vi "THzTime_SPEED_control_TA_170214.vi"(1 "ESP300 Axis":i8=1, 2 "ESP300 Address":string="1", 4 "Lockin Address":string="12") -> ()   [LabVIEW 2010]
panel:
  in  "Axis 1 Step btw Pos":dbl=0.1
  in  "Delay":u32=1500
  in  "?":bool
  in  "# of Avg":i32=8
  in  "Axis 1 # of Pos":u16=40
  in  "Axis 1 Starting Pos":dbl=14.5
  in  "SHOT202 Address":string="8"
  out "Y position":dbl=-0.2690666666666667 format="%#.3p"
  out "X position":dbl=-0.49996666666666667 format="%#.3p"
  out "Power meter":dbl=48.71333333333333 format="%#.3p"
  in  "Save File Name":string="bc_"
  in  "Launch server?":bool
  in  "Authorize?":bool=TRUE
  in  "CONEX-PSD9 Instrument Key 2":string="CONEX-PSD (A6ULD73M)"
  in  "Interdelay (ms)":dbl=20.0
  in  "pre delay(ms)":dbl=300.0
  out "Lock-in Y-Channel":dbl=3.63801e-12 format="%#.3p"
  out "Lock-in X-Channel":dbl=-3.4561e-11 format="%#.3p"
  out "THz Time-domain Signal Wave":cluster{"x-axis":sgl[], "y-axis":dbl[]}(graph)={"x-axis"=[-14.5, -14.51, -14.52, -14.53, -14.54, -14.55, -14.56, -14.57, -14.58, -14.59, -14.6, -14.61], "y-axis"=[1.819e-12, 1.819e-12, 0.0, 0.0, -1.819e-12, -7.27601e-12, -9.095e-12, -1.0914e-11, -1.6371e-11, -2.0009e-11, -2.1828e-11, -2.91041e-11]}
  in  "Autosave Directory for Long-term Average Scan":path=path "D:/taianh/Measurement Data/170219 Beam Calibration"
  in  "OK Button":bool
  out "Data Type":string="outp ? 1"
  in  "Enum":enum16{"X", "Y", "Abs"}(ring)
  in  "Draw":bool
  in  "Exit Program":bool
  in  "Short term \nAverage#":i8=1
  in  "Step":sgl=0.005 min=0 max=10000 format="%.3f"
  in  "End Position":sgl=-8.0 min=-75 max=75 format="%#.3f"
  in  "Start Position":sgl=-6.5 min=-75 max=75 format="%#.3f"
  # "THz Experiment"
  # "Data"
  # "Auto-offset"
  # "Start Position (mm)"
  # "End Position (mm)"
  # "Step (mm)"
  # "Point Avg"
  # "# of Avg"
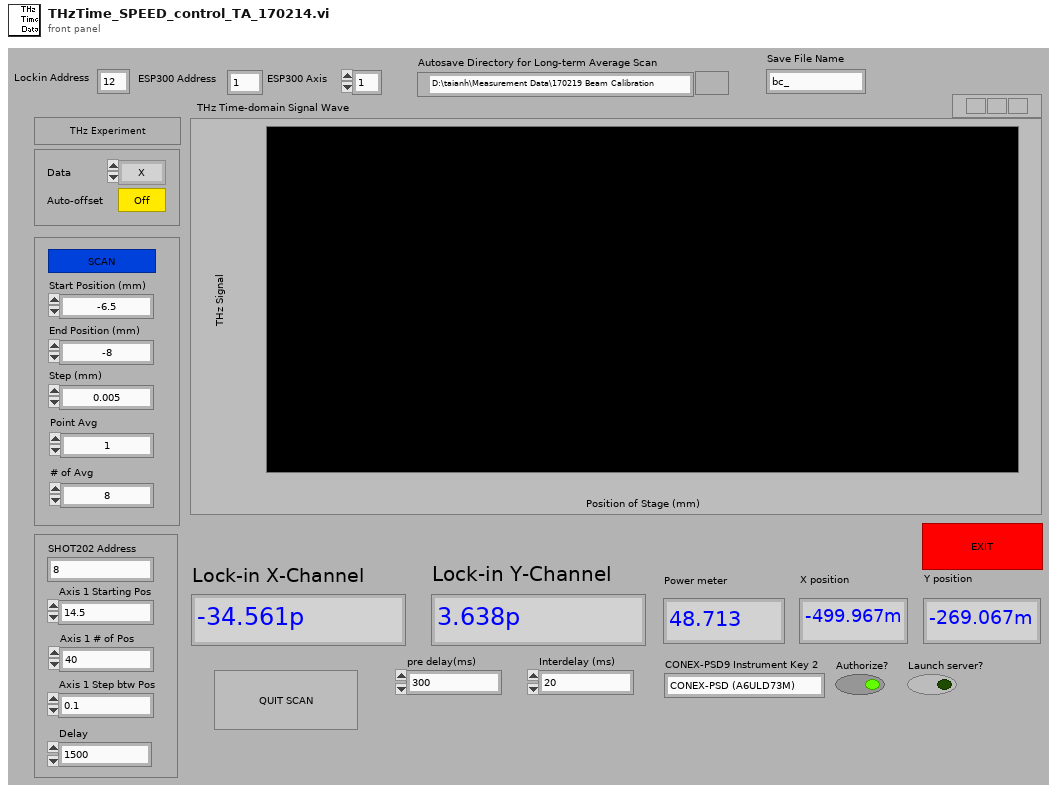
[diagram p1: front panel]
types:
  T1 = cluster{"ConexPSD Reference":refnum<k24>, "error out":errorcluster, "Component ID":i32}
  T2 = cluster{"Step Number":i32, "Step":sgl, "Start Position":sgl, "Time-out":i32, "Lockin Address":string, "Short term \nAverage#":i8, i32, "ESP300 Axis":i8, "Value":string, "pre delay(ms)":dbl, "Interdelay (ms)":dbl, "Autosave Directory for Long-term Average Scan":path, cluster{"ConexPSD Reference":refnum<k24>, "error out":errorcluster, "Component ID":i32}}
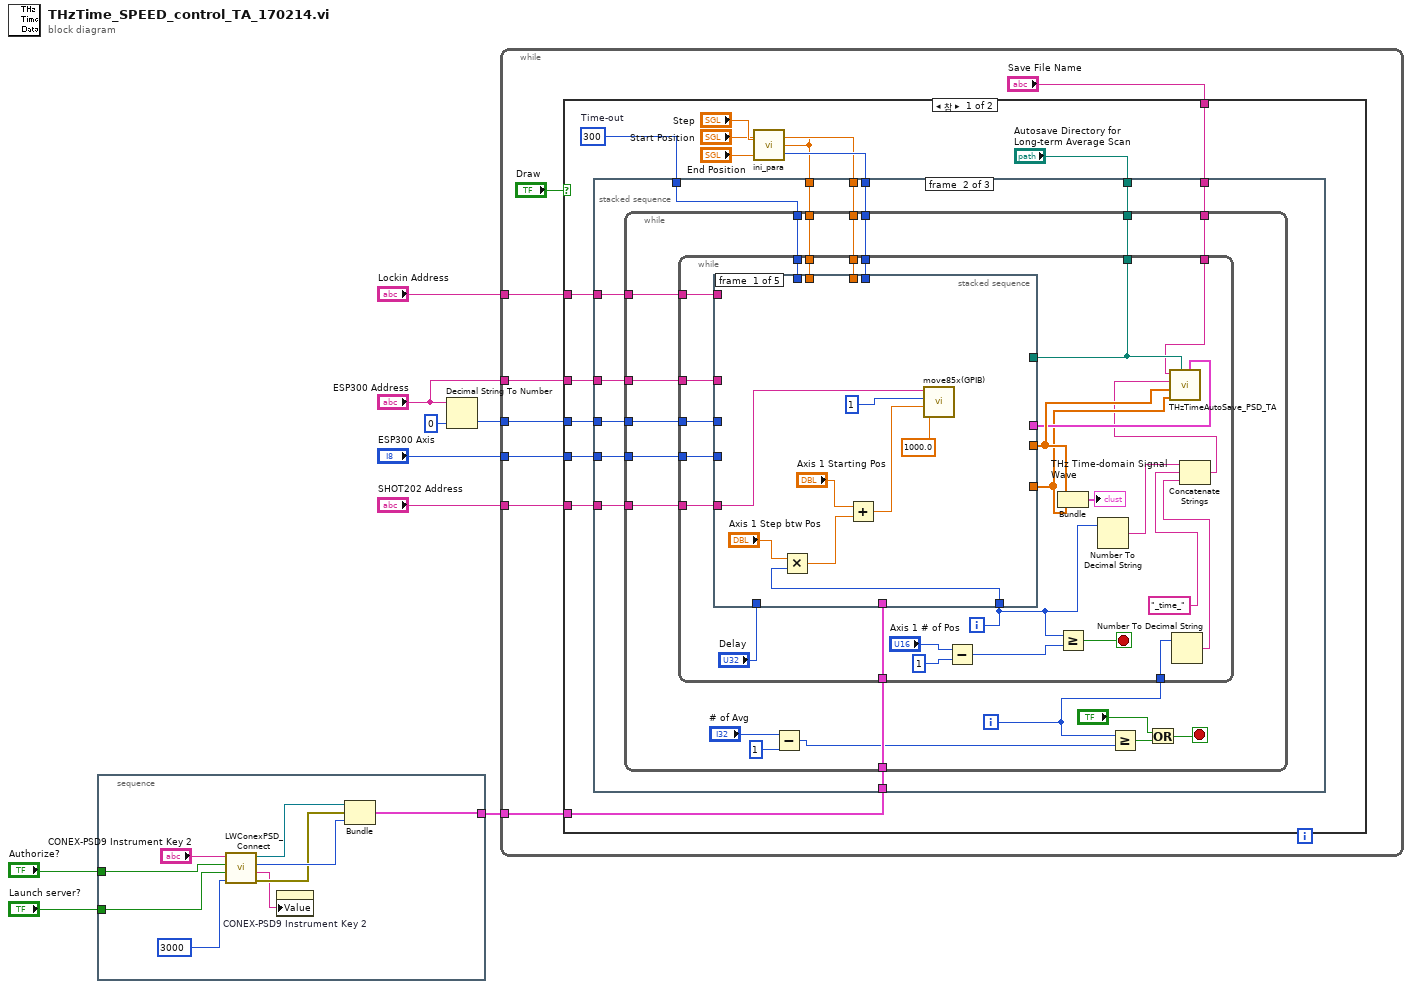
[diagram p0: block diagram]
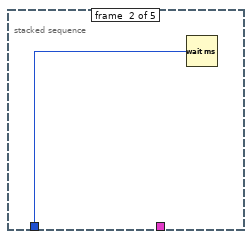
[diagram p3: hidden frame]
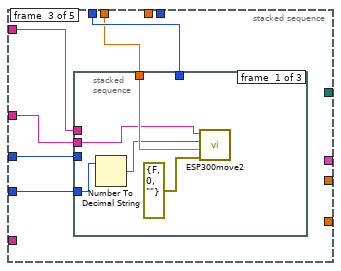
[diagram p4: hidden frame]
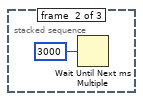
[diagram p5: hidden frame]
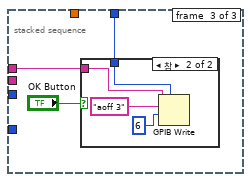
[diagram p6: hidden frame]
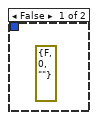
[diagram p7: hidden frame]
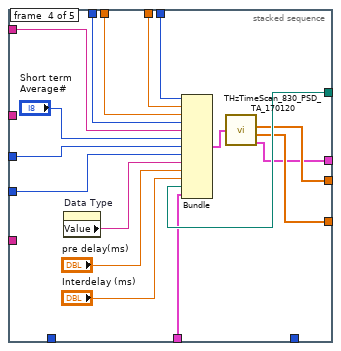
[diagram p8: hidden frame]
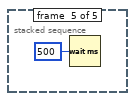
[diagram p9: hidden frame]
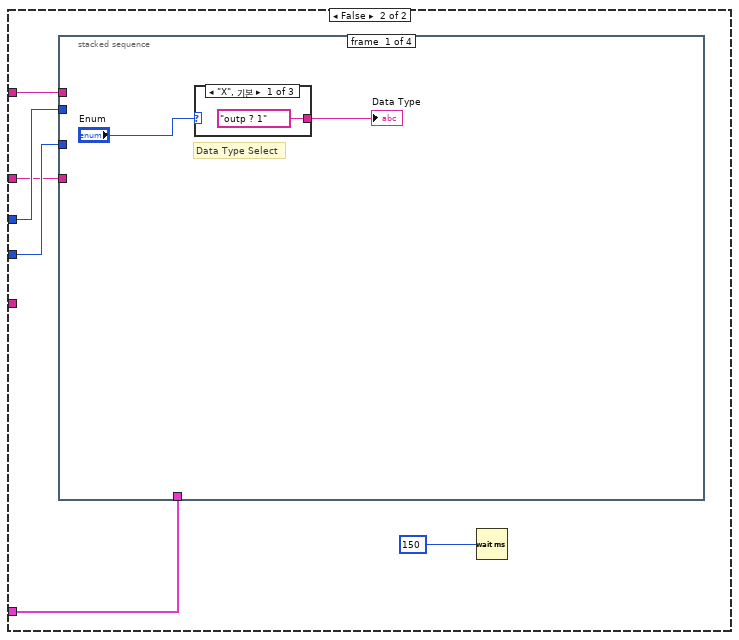
[diagram p11: hidden frame]
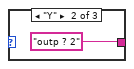
[diagram p12: hidden frame]
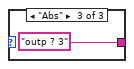
[diagram p13: hidden frame]
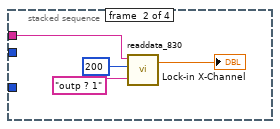
[diagram p14: hidden frame]
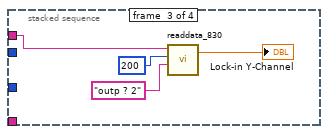
[diagram p15: hidden frame]
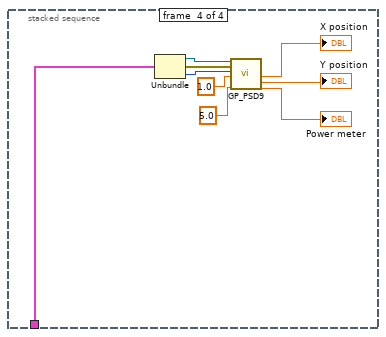
[diagram p16: hidden frame]
diagram:
  n1 = stacked-sequence {
    tunnel: "Authorize?" -> [w12]
    tunnel: [w11] -> w2
    tunnel: "Launch server?" -> [w10]
    frame #0 {
      n2 = call "LWConexPSD_Connect.vi"("DiscoverTimeout (10000 msec)"=3000, "Launch server? (True)"=w10, "Authorize? (True)"=w12, "Instrument Key"="CONEX-PSD9 Instrument Key 2") -> ("error out"=w16:errorcluster, "Instrument Key out"=w14:string, "Component ID"=w17:i32, "ConexPSD Reference"=w15:refnum<k24>)
      n3 = property on="CONEX-PSD9 Instrument Key 2" class="Str"("Value"=w14) -> ()  [unwired: 2 in, 2 out]
      n4 = Bundle("ConexPSD Reference"=w15, "error out"=w16, "Component ID"=w17) -> (w11:T1)  [unwired: 1 in]
    }
  }
  n5 = Decimal String To Number(string="ESP300 Address", default (0L)=0 ("default (0 I32)")) -> (number=w7:i32)  [unwired: 1 in, 1 out]
  n6 = while {
    tunnel: "ESP300 Axis" -> [w25]
    tunnel: "Lockin Address" -> [w24]
    tunnel: w7 -> [w23]
    tunnel: "ESP300 Address" -> [w22]
    tunnel: w2 -> [w21]
    tunnel: "SHOT202 Address" -> [w19]
    stop <- "Exit Program" stop-if-true
    n7 = case shown="참" "Draw" {
      tunnel: w24 -> [w41 w149]
      tunnel: w25 -> [w40 w151]
      tunnel: w23 -> [w39 w150]
      tunnel: w22 -> [w31 w147]
      tunnel: w21 -> [w30 w146]
      tunnel: "Save File Name" -> [w29 _]
      tunnel: w19 -> [w28 _]
      frame True {
        w38 = 300  # Time-out
        n8 = call "ini_para.vi"("End Position"="End Position", "Start Position"="Start Position", "Step"="Step") -> ("Step Number"=w35:i32, "Step"=w34:sgl)
        n9 = stacked-sequence {
          tunnel: w41 -> [_ w53 _]
          tunnel: w38 -> [_ w52 _]
          tunnel: w40 -> [_ w51 _]
          tunnel: w39 -> [_ w50 _]
          tunnel: w35 -> [_ w48 _]
          tunnel: w34 -> [_ w46 _]
          tunnel: "Start Position" -> [_ w49 _]
          tunnel: "Autosave Directory for Long-term Average Scan" -> [_ w47 _]
          tunnel: w31 -> [_ w45 _]
          tunnel: w30 -> [_ w44 _]
          tunnel: w29 -> [_ w43 _]
          tunnel: w28 -> [_ w42 _]
          frame #0 {
          }
          frame #1 {
            n10 = while {
              tunnel: w53 -> [w72]
              tunnel: w52 -> [w71]
              tunnel: w51 -> [w70]
              tunnel: w50 -> [w69]
              tunnel: w49 -> [w68]
              tunnel: w48 -> [w67]
              tunnel: w47 -> [w66]
              tunnel: w46 -> [w65]
              tunnel: w45 -> [w64]
              tunnel: w44 -> [w63]
              tunnel: w43 -> [w62]
              tunnel: w42 -> [w61]
              i -> [w54]
              stop <- w56 stop-if-true
              n11 = while {
                tunnel: w71 -> [w98]
                tunnel: w72 -> [w99]
                tunnel: w70 -> [w97]
                tunnel: w69 -> [w96]
                tunnel: w68 -> [w95]
                tunnel: w65 -> [w94]
                tunnel: w67 -> [w93]
                tunnel: w66 -> [w88]
                tunnel: w64 -> [w91]
                tunnel: w63 -> [w90]
                tunnel: w62 -> [w87]
                tunnel: w61 -> [w84]
                tunnel: w54 -> [w75]
                i -> [w78]
                stop <- w83 stop-if-true
                n12 = stacked-sequence {
                  tunnel: w99 -> [_ _ w114 w140 _]
                  tunnel: w98 -> [_ _ w113 w141 _]
                  tunnel: w97 -> [_ _ w112 w137 _]
                  tunnel: w96 -> [_ _ w111 w138 _]
                  tunnel: w95 -> [_ _ w110 w142 _]
                  tunnel: w94 -> [_ _ _ w143 _]
                  tunnel: w93 -> [_ _ _ w144 _]
                  tunnel: [_ _ _ w131 _] -> w89
                  tunnel: [_ _ _ w130 _] -> w85
                  tunnel: w91 -> [_ _ w109 _ _]
                  tunnel: w88 -> [_ _ _ w133 _]
                  tunnel: w90 -> [_ _ _ w132 _]
                  tunnel: [_ _ _ w129 _] -> w86
                  tunnel: w84 -> [w107 _ _ _ _]
                  tunnel: w78 -> [w105 _ _ _ _]
                  tunnel: "Delay" -> [_ w108 _ _ _]
                  frame #0 {
                    n13 = Multiply(x="Axis 1 Step btw Pos", y=w105) -> (x*y=w102:dbl)
                    n14 = Add(x="Axis 1 Starting Pos", y=w102) -> (x+y=w101:dbl)
                    n15 = call "move85x(GPIB).vi"("wait time(ms)"=1000.0, "Moving Distance (mm) : resolutino is 1um"=w101, "Axis Number"=u8 1, "SHOT202 Address"=w107) -> ()
                  }
                  frame #1 {
                    n16 = Wait (ms)(milliseconds to wait=w108) -> ()  [unwired: 1 out]
                  }
                  frame #2 {
                    n17 = stacked-sequence {
                      tunnel: w114 -> [_ _ w122]
                      tunnel: w113 -> [_ _ w121]
                      tunnel: w112 -> [w116 _ _]
                      tunnel: w111 -> [_ _ _]
                      tunnel: w110 -> [w119 _ _]
                      tunnel: w109 -> [w117 _ _]
                      frame #0 {
                        n18 = Number To Decimal String(number=w116) -> (decimal integer string=w115:string)  [unwired: 1 in]
                        n19 = call "ESP300move2.vi"("ESP300 Address"=w117, "ESP300 Channel"=w115, "Target"=w119, "error in (no error) 2"=errorcluster {"status"=FALSE, "code"=0, "source"=""}) -> ()  [unwired: 6 in, 1 out]
                      }
                      frame #1 {
                        n20 = Wait Until Next ms Multiple(millisecond multiple=3000) -> ()  [unwired: 1 out]
                      }
                      frame #2 {
                        n21 = case shown="참" "OK Button" {
                          tunnel: w122 -> [_ w127]
                          tunnel: w121 -> [_ w125]
                          frame False {
                            (unwired) errorcluster {"status"=FALSE, "code"=0, "source"=""} ("error in")
                          }
                          frame True {
                            n22 = GPIB Write(0:w127, 1:"aoff 3" ("data"), 2:i16 6 ("mode (0)"), 4:w125) -> ()  [unwired: 1 in, 2 out]
                          }
                        }
                      }
                    }
                  }
                  frame #3 {
                    n23 = property on="Data Type" class="Str"() -> ("Value"=w136:string)  [unwired: 2 in, 2 out]
                    n24 = Bundle("Step Number"=w144, "Step"=w143, "Start Position"=w142, "Time-out"=w141, "Lockin Address"=w140, "Short term \nAverage#"="Short term \nAverage#", w138, "ESP300 Axis"=w137, "Value"=w136, "pre delay(ms)"="pre delay(ms)", "Interdelay (ms)"="Interdelay (ms)", "Autosave Directory for Long-term Average Scan"=w133, w132) -> (w128:T2)  [unwired: 1 in]
                    n25 = call "THzTimeScan_830_PSD_TA_170120.vi"("input"=w128) -> ("x-axis"=w131:sgl[], "y-axis"=w130:dbl[], "ext. out"=w129:cluster{dbl[], dbl[], dbl[], dbl[], string[]})  [unwired: 1 out]
                  }
                  frame #4 {
                    n26 = Wait (ms)(milliseconds to wait=u32 500) -> ()  [unwired: 1 out]
                  }
                }
                n27 = Subtract(x="Axis 1 # of Pos", y=u16 1) -> (x-y=w79:u16)
                n28 = Bundle("x-axis"=w89, "y-axis"=w85) -> (→"THz Time-domain Signal Wave":cluster{"x-axis":sgl[], "y-axis":dbl[]})  [unwired: 1 in]
                n29 = Greater Or Equal?(x=w78, y=w79) -> (x >= y?=w83:bool)
                n30 = Number To Decimal String(number=w78) -> (decimal integer string=w73:string)  [unwired: 1 in]
                n31 = Number To Decimal String(number=w75) -> (decimal integer string=w74:string)  [unwired: 1 in]
                n32 = Concatenate Strings(w73, "_time_", w74) -> (w77:string)
                n33 = call "THzTimeAutoSave_PSD_TA.vi"("ext. out"=w86, "Autosave Directory for Long-term Average Scan"=w88, "y-axis"=w85, "x-axis"=w89, "String"=w77, "SaveFile name"=w87) -> ()  [unwired: 4 in]
              }
              n34 = Subtract(x="# of Avg", y=1) -> (x-y=w55:i32)
              n35 = Greater Or Equal?(x=w54, y=w55) -> (x >= y?=w58:bool)
              n36 = Or(x="?", y=w58) -> (x .or. y?=w56:bool)
            }
          }
          frame #2 {
          }
        }
      }
      frame False {
        n37 = stacked-sequence {
          tunnel: w151 -> [_ _ _ _]
          tunnel: w150 -> [_ _ _ _]
          tunnel: w149 -> [_ w160 w164 _]
          tunnel: w147 -> [_ _ _ _]
          tunnel: w146 -> [_ _ _ w165]
          frame #0 {
            # "Data Type Select"
            n38 = case shown="\"X\", 기본" "Enum" {
              tunnel: ["outp ? 1" "outp ? 2" "outp ? 3"] -> w153
              frame "X", Default {
              }
              frame "Y" {
              }
              frame "Abs" {
              }
            }
            "Data Type" <- w153
          }
          frame #1 {
            n39 = call "readdata_830.vi"("Command"="outp ? 1", "timeout"=200, "Lockin Address"=w160) -> ("Data"=→"Lock-in X-Channel":dbl)  [unwired: 1 in, 1 out]
          }
          frame #2 {
            n40 = call "readdata_830.vi"("Command"="outp ? 2", "timeout"=200, "Lockin Address"=w164) -> ("Data"=→"Lock-in Y-Channel":dbl)  [unwired: 1 in, 1 out]
          }
          frame #3 {
            n41 = Unbundle(w165) -> ("ConexPSD Reference"=w173:refnum<k24>, "error out"=w172:errorcluster, "Component ID"=w171:i32)
            n42 = call "GP_PSD9.vi"("ConexPSD Reference"=w173, "error out"=w172, "Component ID"=w171, "Adress"=1.0 ("shot average"), "shot average"=5.0) -> ("PositionX"=→"X position":dbl, "PositionY"=→"Y position":dbl, "LaserPower"=→"Power meter":dbl)  [unwired: 8 in, 4 out]
          }
        }
        n43 = Wait (ms)(milliseconds to wait=u32 150) -> ()  [unwired: 1 out]
      }
    }
  }
